vi "solar Refnum Type Cast (Preview).vi"(2 "Refnum":T5, 3 "Timeout in ms (-1)":i32=-1) -> (7 "SOLAR":T1)   [LabVIEW 2018]
doc: "This type casts the solar reference and returns the value of the solar data."
uses:
  solar_ctl Target Global.ctl
  solar_ctl SOLAR Global.ctl
  voyager/solar_voy_ctl Voyager Refnum.ctl
  qtimer/solar_qtimer_ctl Refnum.ctl
  solar_ctl SOLAR Refnum.ctl
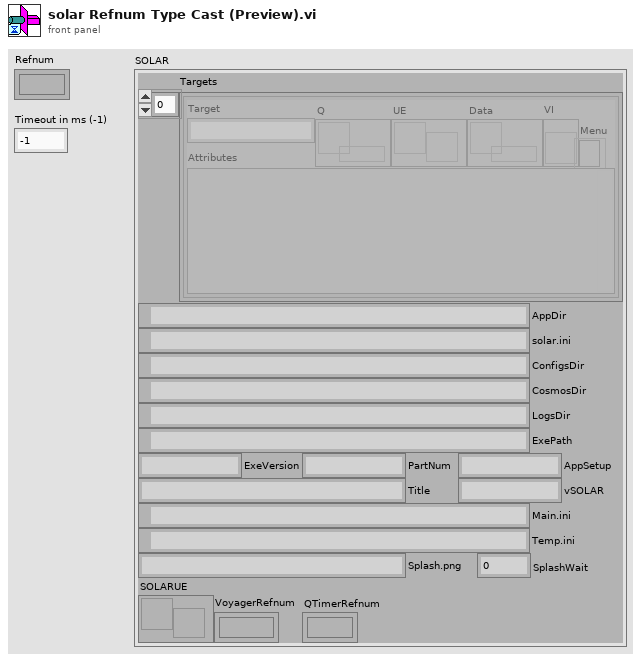
[diagram p1: front panel]
types:
  T1 = typedef "solar_ctl SOLAR Global.ctl" = cluster{"Targets":T2[], "AppDir":path, "solar.ini":path, "ConfigsDir":path, "CosmosDir":path, "LogsDir":path, "ExePath":path, "ExeVersion":string, "PartNum":string, "AppSetup":string, "Title":string, "Main.ini":path, "Temp.ini":path, "vSOLAR":string, "Splash.png":string, "SplashWait":i32, "SOLARUE":refnum<user-event>, "VoyagerRefnum":T3, "QTimerRefnum":T4}
  T2 = typedef "solar_ctl Target Global.ctl" = cluster{"Target":string, "Q":refnum<queue>, "UE":refnum<user-event>, "VI":refnum<vi>, "Menu":refnum<k9>, "Data":refnum<data-value>, "Attributes":variant}
  T3 = typedef "solar_voy_ctl Voyager Refnum.ctl" = refnum<k1>
  T4 = typedef "solar_qtimer_ctl Refnum.ctl" = refnum<k1>
  T5 = typedef "solar_ctl SOLAR Refnum.ctl" = refnum<k1>
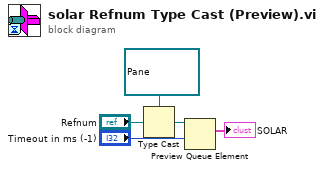
[diagram p0: block diagram]
diagram:
  n1 = Type Cast(type=refnum<queue> refnum ("SOLAR"), x="Refnum") -> (*(type *) &x=w4:refnum<queue>)
  n2 = Preview Queue Element(queue=w4, timeout in ms (-1)="Timeout in ms (-1)") -> (element=→"SOLAR":T1)  [unwired: 1 in, 3 out]
